vi "HXQ-钩外多胶-检测.vi"(5 "裁切偏移":i32[](array[numeric]), 7 "ImgRef":T8(plugin-control), 9 "MirroredAngle":dbl, 10 "Global Rectangle":i32[](array[numeric]), 11 "ImageSRC":T8(plugin-control)) -> (0 "顶洞缺胶状态正常":bool, 1 "多胶异常RECT":cluster{dbl, dbl, dbl, dbl}, 2 "钩外多胶正常":bool, 3 "ImageOUT":T8(plugin-control))   [LabVIEW 2018]
uses:
  <vilib>/vision/Measure.llb/Straight Edge Options.ctl
  <vilib>/vision/Measure.llb/Straight Edge Process.ctl
  <vilib>/vision/Measure.llb/Edge Options.ctl
  <vilib>/vision/Measure.llb/Edge Polarity.ctl
  <vilib>/vision/Image Controls.llb/IMAQ Image.ctl
  <vilib>/vision/Contour.llb/IMAQ Contour Curve Extraction.ctl
  <vilib>/Analysis/coordinate.llb/Angle Units.ctl
  <vilib>/Analysis/coordinate.llb/Check for Included Angle (scalar).vi
  <vilib>/Analysis/coordinate.llb/Wrap Angle (scalar).vi
  <vilib>/Analysis/coordinate.llb/Absolute Angle Difference (scalar).vi
  <vilib>/Analysis/coordinate.llb/Set Angle Unit.vi
  <vilib>/vision/NI_Vision_Development_Module.lvlib
  <vilib>/Analysis/NI_AAL_Angle.lvlib
  <vilib>/vision/Contour.llb/IMAQ Connect Range Setting.ctl
panel:
  in  "Contour Points Settings":T1={"Overlay?"=TRUE, "Color"=16738816, "Width"=1, "Maintain Width?"=TRUE}
  in  "Kernel Width":u32=31
  in  "Curve Extraction Settings":T2={"Extraction Mode"=0, "Edge Threshold"=30, "Edge Filter Size"=2, "Min Length"=10, "Search Step Size"=10, "Max Endpoint Gap"=20, "Subpixel"=TRUE} {"Extraction Mode" items=["Normal", "Uniform Regions"]; "Edge Filter Size" items=["Fine", "Normal", "Contour Tracing"]; "Max Endpoint Gap" min=0; "Search Step Size" min=1 max=255 step=1; "Min Length" min=0; "Edge Threshold" min=1 max=350 step=1}
  out "Curvature Profile":dbl[](graph)
  in  "顶洞_RakeEdge Options 2":T3={"Edge Polarity"=0, "Kernel Size"=3, "Width"=9, "Minimum Edge Strength"=50.0, "Interpolation Type"=enum."Bilinear Fixed", "Data Processing Method"=enum."Average"} {"Edge Polarity" items=["All Edges", "Rising Edges", "Falling Edges"]; "Minimum Edge Strength" format="%.2f"; "Width" step=2; "Kernel Size" step=2}
  out "顶洞圆半径正常":bool
  out "顶洞圆半径":dbl
  in  "顶洞圆半径下限":dbl=50.0
  in  "顶洞圆半径上限":dbl=330.0
  out "Fitted Circle":T5 {"Average SNR (dB)" format="%.2f"; "Average Strength" format="%.2f"; "Roundness (Real-World)" format="%.2f"; "Radius (Real-World)" format="%.2f"; "Center (Real-World)"."Y" format="%.2f"; "Center (Real-World)"."X" format="%.2f"; "Radius (Pixels)" format="%.2f"; "Center (Pixels)"."Y" format="%.2f"; "Center (Pixels)"."X" format="%.2f"}
  in  "顶洞_Options":T6={"Search  Direction"=0, "Edge Options"={"Edge Polarity"=0, "Kernel Size"=3, "Width"=9, "Minimum Edge Strength"=50.0, "Interpolation Type"=enum."Bilinear Fixed", "Data Processing Method"=enum."Average"}, "Show Search Area"=TRUE, "Show Search Lines"=FALSE, "Show Edges Found"=FALSE, "Show Result"=TRUE, "Search Area Color"=65280, "Search Lines Color"=255, "Edge Locations Color"=16776960, "Result Color"=16711680, "Overlay Group Name"=""} {"Search  Direction" items=["Outside to Inside", "Inside to Outside"]; "Edge Options"."Edge Polarity" items=["All Edges", "Rising Edges", "Falling Edges"]; "Edge Options"."Minimum Edge Strength" format="%.2f"; "Edge Options"."Width" step=2; "Edge Options"."Kernel Size" step=2}
  in  "顶洞_Circle Fit Options":T7={"Process"=enum."Get First Edge", "Step Size"=3.0, "Max Pixel Radius"=3}
  in  "ROI_顶洞检测扇形半张角":dbl=17.0 format="%#_13g"
  in  "R_顶洞检测小圆半径":i32=136
  out "ImgOut":T8(plugin-control)
  in  "偏移_顶洞_向上部修正量":dbl=230.0 format="%#_13g"
  in  "槽宽比例限度":dbl=0.04
  out "多胶异常RECT本地":T9
  out "error out 2":errorcluster
  out "Image Out":T8
  in  "偏移_钩端_向上部修正量":dbl=209.0 format="%#_13g"
  in  "初始ROI下行参数":dbl=1.0
  in  "高径比参数值":dbl=0.6
  out "边沿检测LineProfile原始":dbl[](graph)
  out "波形2":dbl[](graph) caption="Line Profile"
  out "边沿检测梯度":dbl[](graph)
  in  "溢槽槽向边沿检测":T3={"Edge Polarity"=1, "Kernel Size"=7, "Width"=37, "Minimum Edge Strength"=50.0, "Interpolation Type"=enum."Bilinear Fixed", "Data Processing Method"=enum."Average"} {"Edge Polarity" items=["All Edges", "Rising Edges", "Falling Edges"]; "Minimum Edge Strength" format="%.2f"; "Width" step=2; "Kernel Size" step=2}
  out "所得中线的端点属于正序":bool caption="范围内？"
  out "Angles (deg)":sgl[](array[numeric]) format="%.2f"
  out "error out":errorcluster
  in  "error in (no error)":errorcluster
  in  "Image":T8
  in  "Edge Options横向槽边":T3={"Edge Polarity"=2, "Kernel Size"=7, "Width"=13, "Minimum Edge Strength"=70.0, "Interpolation Type"=enum."Bilinear Fixed", "Data Processing Method"=enum."Average"} {"Edge Polarity" items=["All Edges", "Rising Edges", "Falling Edges"]; "Minimum Edge Strength" format="%.2f"; "Width" step=2; "Kernel Size" step=2}
  in  "Line Options":T10={"Number of Lines"=1, "Type"=enum."First Edge Rake", "Min. Score"=100.0, "Max. Score"=1000.0, "Orientation"=0.0, "Angle Range"=10.0, "Angle Tolerance"=1.0, "Step Size"=5, "Min. SNR (db)"=0.0, "Min. Points (%)"=25.0, "Hough Iterations"=5} {"Min. Points (%)" min=0.0 max=100.0; "Min. SNR (db)" min=0.0; "Max. Score" min=0.0 max=1024.0; "Min. Score" min=0.0 max=1024.0 step=1.0}
  # "小洞，大洞：50,110"
  # "进行槽的横向边沿检测的时候\n最好对强度阈值进行动态自动配置，避免定值"
  # "槽的边沿强度需要认真设定，避免强度门槛太低引入干扰致找错位置。"
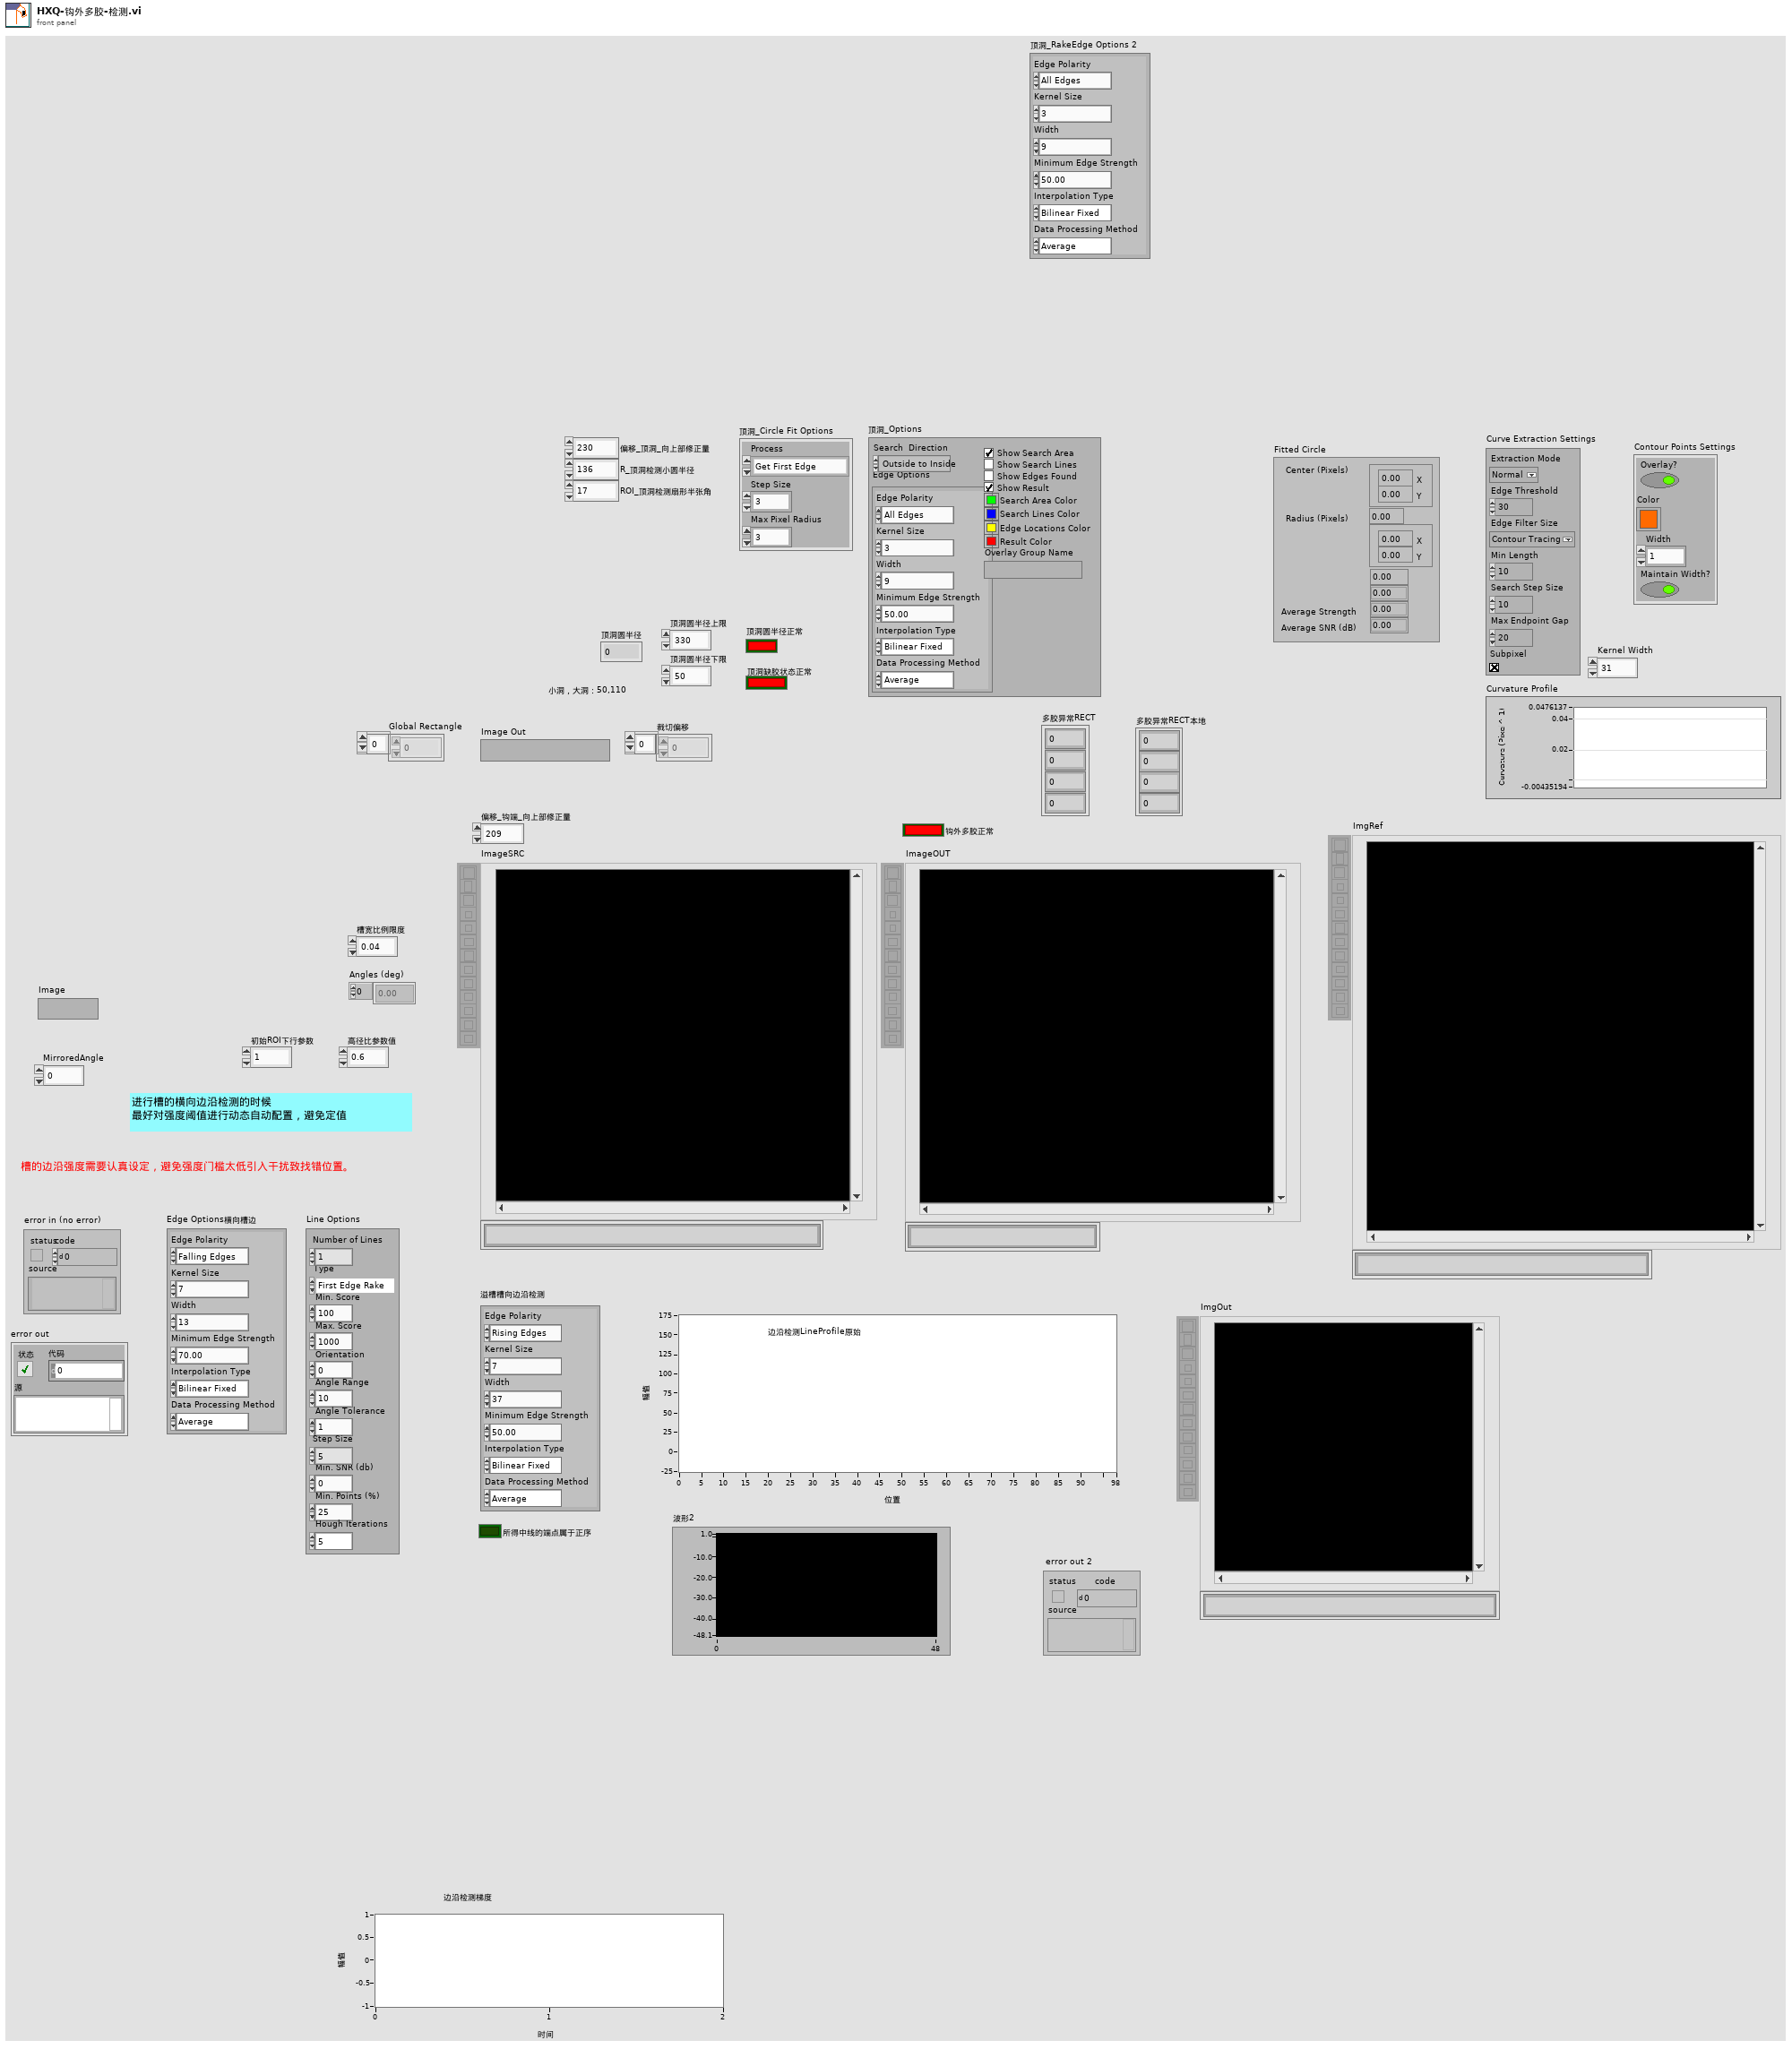
[diagram p1: front panel]
types:
  T1 = cluster{"Overlay?":bool, "Color":u32, "Width":u32, "Maintain Width?":bool}
  T2 = typedef "IMAQ Contour Curve Extraction.ctl" = cluster{"Extraction Mode":u32, "Edge Threshold":i32, "Edge Filter Size":u32, "Min Length":i32, "Search Step Size":i32, "Max Endpoint Gap":i32, "Subpixel":bool}
  T3 = typedef "Edge Options.ctl" = cluster{"Edge Polarity":T4, "Kernel Size":u32, "Width":u32, "Minimum Edge Strength":sgl, "Interpolation Type":enum32{"Zero Order", "Bilinear", "Quadratic", "Cubic", "Bilinear Fixed"}, "Data Processing Method":enum32{"Average", "Median"}}
  T4 = typedef "Edge Polarity.ctl" = u32
  T5 = cluster{"Center (Pixels)":cluster{"X":sgl, "Y":sgl}, "Radius (Pixels)":dbl, "Center (Real-World)":cluster{"X":sgl, "Y":sgl}, "Radius (Real-World)":dbl, "Roundness (Real-World)":dbl, "Average Strength":dbl, "Average SNR (dB)":dbl}
  T6 = cluster{"Search  Direction":u32, "Edge Options":T3, "Show Search Area":bool, "Show Search Lines":bool, "Show Edges Found":bool, "Show Result":bool, "Search Area Color":u32, "Search Lines Color":u32, "Edge Locations Color":u32, "Result Color":u32, "Overlay Group Name":string}
  T7 = cluster{"Process":enum16{"Get First Edge", "Get First + Last Edge", "Get All Edges", "Get Best Edge"}, "Step Size":dbl, "Max Pixel Radius":i32}
  T8 = typedef "IMAQ Image.ctl" = refnum<image>
  T9 = cluster{"Numeric":dbl, "Numeric":dbl, "Numeric":dbl, "Numeric":dbl}
  T10 = typedef "Straight Edge Options.ctl" = cluster{"Number of Lines":i32, "Type":T11, "Min. Score":dbl, "Max. Score":dbl, "Orientation":dbl, "Angle Range":dbl, "Angle Tolerance":dbl, "Step Size":u32, "Min. SNR (db)":dbl, "Min. Points (%)":dbl, "Hough Iterations":i32}
  T11 = typedef "Straight Edge Process.ctl" = enum32{"First Edge Rake", "Best Edge Rake", "Hough Edge Rake", "First Edge Projection", "Best Edge Projection"}
  T12 = typedef "IMAQ Point" = cluster{"X":sgl, "Y":sgl}
  T13 = enum16{"Get First Edge", "Get First + Last Edge", "Get All Edges", "Get Best Edge"}
  T14 = typedef "ROI Descriptor" = cluster{"Global Rectangle":i32[], "Contours":cluster{"ID":enum32{"External", "Internal"}, "Type":u32, "Coordinates":i32[]}[]}
  T15 = cluster{"X":dbl, "Y":dbl, "X":dbl, "Y":dbl, "Height":dbl}
  T16 = typedef "Edge New.ctl" = cluster{"Location (Pixel)":cluster{"X":sgl, "Y":sgl}, "Location (Real-World)":cluster{"X":sgl, "Y":sgl}, "Distance (Pixel)":dbl, "Distance (Real-World)":dbl, "Strength":dbl, "Noise":dbl, "Rising?":bool}
  T17 = typedef "Search Line.ctl" = cluster{"Start Point":cluster{"X":sgl, "Y":sgl}, "End Point":cluster{"X":sgl, "Y":sgl}, "Edge Info":T16[], "Edge Map":dbl[], "Calibration Valid":bool}
  T18 = cluster{"Point1 (Pixels)":cluster{"X":sgl, "Y":sgl}, "Point2 (Pixels)":cluster{"X":sgl, "Y":sgl}, "Point1 (Real-World)":cluster{"X":sgl, "Y":sgl}, "Point2 (Real-World)":cluster{"X":sgl, "Y":sgl}, "Angle (Pixel)":dbl, "Angle (Real-World)":dbl, "Score":dbl, "Straightness":dbl, "Average SNR (db)":dbl, "Calibration Valid":bool}[]
  T19 = cluster{"Point1 (Pixels)":cluster{"X":sgl, "Y":sgl}, "Point2 (Pixels)":cluster{"X":sgl, "Y":sgl}, "Point1 (Real-World)":cluster{"X":sgl, "Y":sgl}, "Point2 (Real-World)":cluster{"X":sgl, "Y":sgl}, "Angle (Pixel)":dbl, "Angle (Real-World)":dbl, "Score":dbl, "Straightness":dbl, "Average SNR (db)":dbl, "Calibration Valid":bool}
  T20 = cluster{"Point2 (Pixels)":cluster{"X":sgl, "Y":sgl}, "Point1 (Pixels)":cluster{"X":sgl, "Y":sgl}}
  T21 = typedef "IMAQ Line" = cluster{"Start X":i32, "Start Y":i32, "End X":i32, "End Y":i32}
  T22 = typedef "IMAQ Circle" = cluster{"Center X":i32, "Center Y":i32, "Inner Radius":i32, "Outer Radius":i32, "Start Angle":dbl, "End Angle":dbl}
  T23 = typedef "IMAQ Connect Range Setting.ctl" = cluster{"Match Constraints":u32, "Min":dbl, "Max":dbl}
  T24 = enum16{"Closest To Search Start", "Maximum Length", "Strongest Mean Gradient Change"}
  T25 = enum16{"Rect Left To Right", "Rect Right To Left", "Rect Top To Bottom", "Rect Bottom To Top", "Annulus Inner To Outer", "Annulus Outer To Inner", "Annulus Start Angle To End Angle", "Annulus End Angle To Start Angle"}
  T26 = typedef "IMAQ Rectangle" = cluster{"Left":i32, "Top":i32, "Right":i32, "Bottom":i32, "Rotation":dbl}
  T27 = typedef "NI_AAL_Angle.lvlib/Angle Units.ctl" = i32
  T28 = cluster{"Point1 (Pixels)":cluster{"X":sgl, "Y":sgl}, "Point2 (Pixels)":cluster{"X":sgl, "Y":sgl}}
  T29 = cluster{"Point 1":cluster{"X":sgl, "Y":sgl}, "Point 2":cluster{"X":sgl, "Y":sgl}}
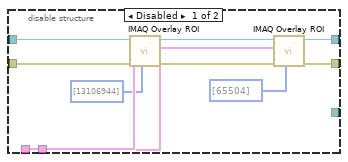
[diagram p4: hidden frame]
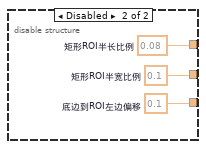
[diagram p5: hidden frame]
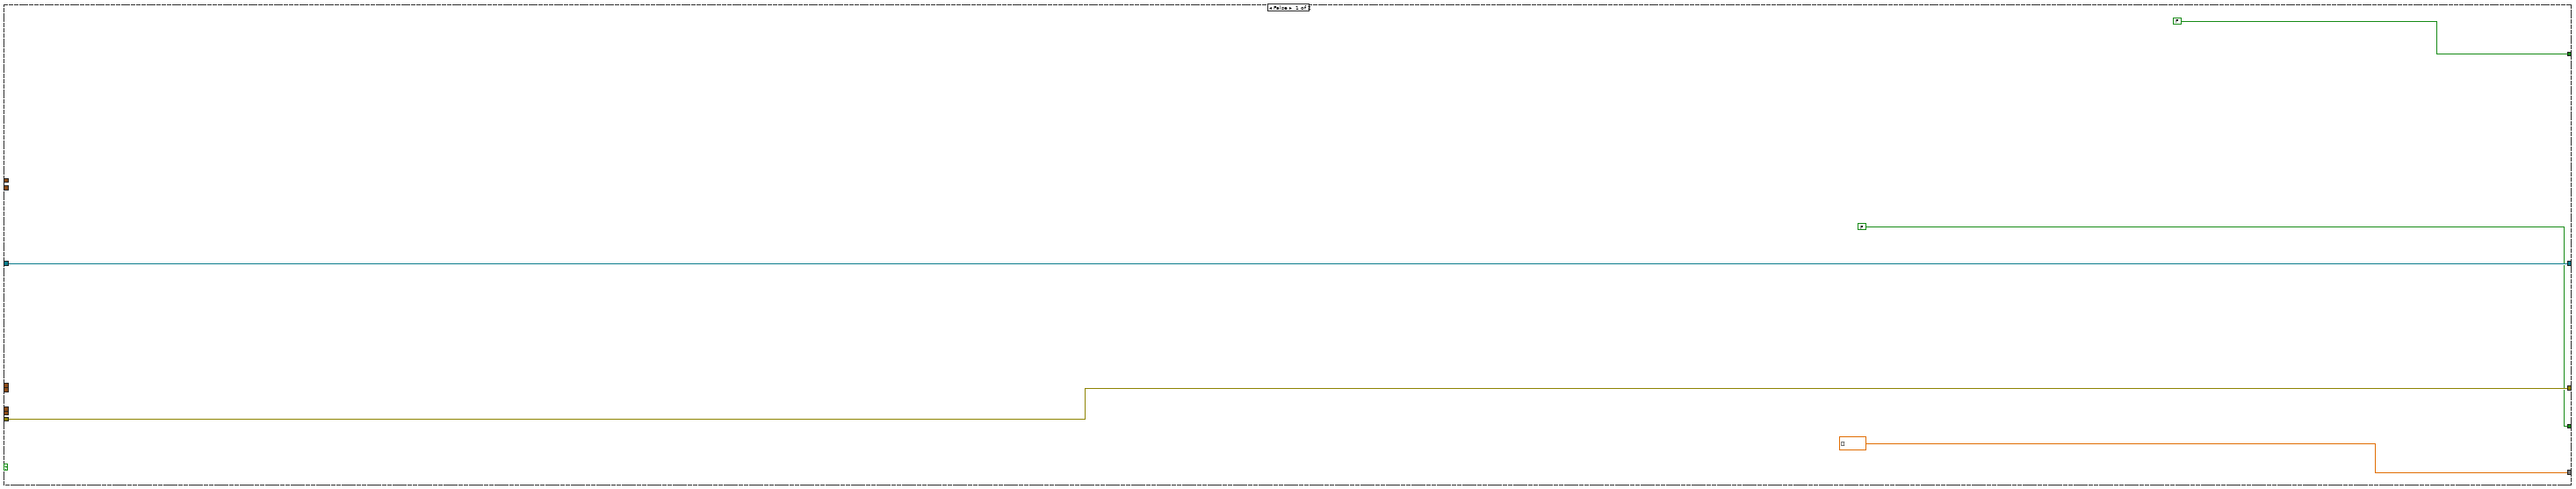
[diagram p13: hidden frame]
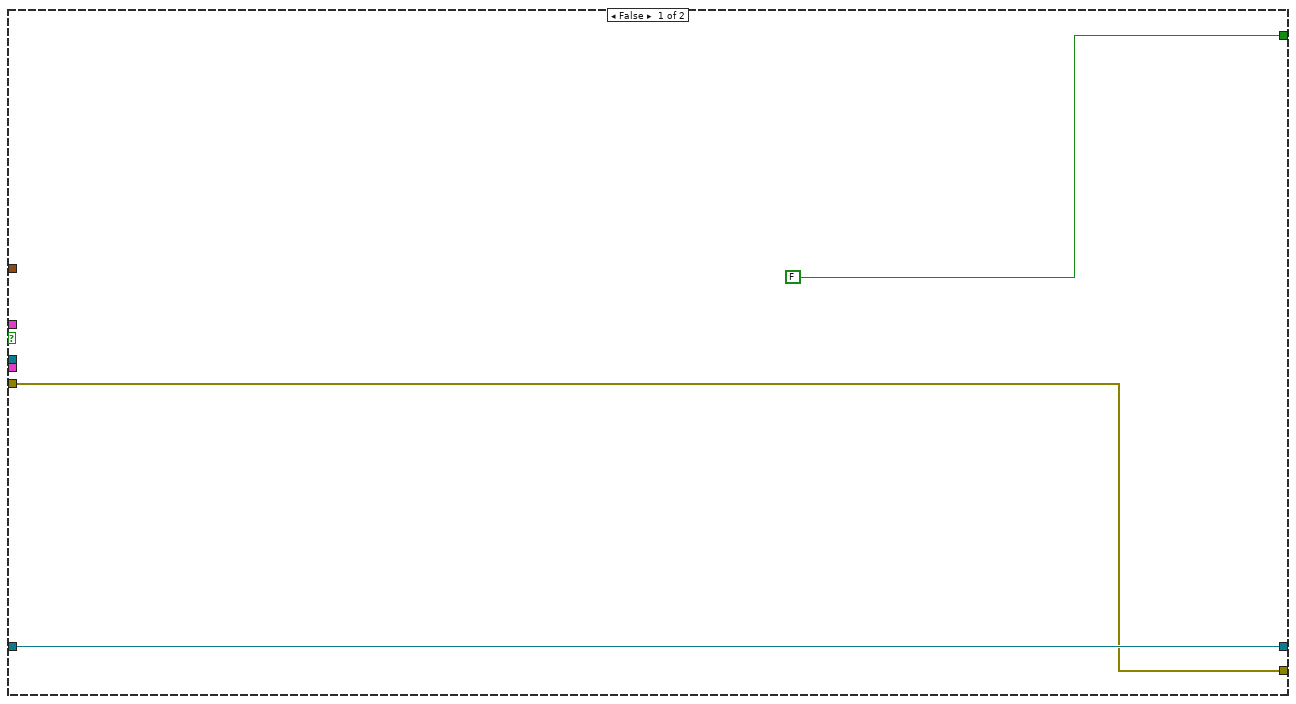
[diagram p14: hidden frame]
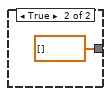
[diagram p19: hidden frame]
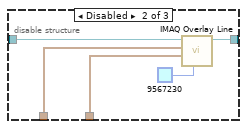
[diagram p20: hidden frame]
diagram:
  w1 = TRUE ("顶洞缺胶状态正常")
  w68 = T12 {"X"=0.5, "Y"=0.5}  # 中点比例
  w83 = 0.1  # 底边到ROI左边偏移
  w81 = 0.15  # 矩形ROI半宽比例
  w80 = 0.05  # 矩形ROI半长比例
  w88 = 0.5 ("y")
  w143 = 0.5 ("y")
  w124 = -0.05  # 底边到ROI左边偏移
  w123 = 0.03  # 矩形ROI半宽比例
  w122 = 0.1  # 矩形ROI半长比例
  # "获取槽位的边沿强度，\n用以指导随后的边线搜索时边沿强度阈值"
  # "经验值"
  # "注意：如果外部裁切时遇到边界，则裁切的XY尺寸会发生异常，\n不能代表产品的半径，导致定位异常。"
  # "构建ROI用于检测铜底最低点"
  # "找寻铜底最低处的位置\n给出准确的基准用于划定扇形ROI选出钩端区域"
  # "从大图中截取时，适当留出边际，以免检测底沿时遇到图像边界。"
  # "矩形ROI的大小，最好改为与底圆直径挂钩，以免后期调节（已挂钩）"
  n1 = disable-structure shown="启用" {
    disable-tunnel: [w169 w172] -> w163
    disable-tunnel: [w168 w171] -> w162
    disable-tunnel: [w167 w170] -> w161
    frame Enabled {
      w167 = 0.06  # 底边到ROI左边偏移
      w168 = 0.11  # 矩形ROI半宽比例
      w169 = 0.15  # 矩形ROI半长比例
    }
    frame Disabled {
      w170 = 0.1  # 底边到ROI左边偏移
      w171 = 0.1  # 矩形ROI半宽比例
      w172 = 0.08  # 矩形ROI半长比例
    }
  }
  n2 = call "IMAQ Clear Overlay"("Image"="ImgRef") -> ("error out"=w125:errorcluster, "Image Out"=w115:T8)  [unwired: 9 in]
  n3 = call "IMAQ GetImageSize"("Image"=w115, "error in (no error)"=w125) -> ("Y Resolution"=w129:i32, "X Resolution"=w130:i32, "error out"=w128:errorcluster)  [unwired: 2 in]
  n4 = Multiply(x=w130, y=w143) -> (x*y=w140:dbl)
  n5 = Multiply(x=w129, y=w143) -> (x*y=w144:dbl)
  n6 = call "IMAQ GetImageSize"("Image"="ImageSRC", "error in (no error)"="error in (no error)") -> ("Y Resolution"=w84:i32, "X Resolution"=w33:i32, "error out"=w27:errorcluster)  [unwired: 2 in]
  n7 = call "HXQ-局部-创建特征检测矩形区域A.vi"("方向角"="MirroredAngle", "产品参考半径"=w33, "底边到ROI左边偏移"=w161, "高径比参数值"="高径比参数值", "矩形ROI半宽比例"=w162, "矩形ROI半长比例"=w163, "Y Resolution"=w84, "X Resolution"=w33) -> ("矩形输出"=w17:cluster{dbl, dbl, dbl, dbl, dbl})  [unwired: 1 in, 2 out]
  n8 = Bundle(w140, w144) -> (w142:cluster{dbl, dbl})  [unwired: 1 in]
  n9 = call "HXQ-局部-创建特征检测矩形区域A.vi"("方向角"="MirroredAngle", "产品参考半径"=w33, "底边到ROI左边偏移"=w83, "矩形ROI半宽比例"=w81, "矩形ROI半长比例"=w80, "Y Resolution"=w84, "X Resolution"=w33) -> ("Height"=w47:dbl, "矩形输出"=w79:cluster{dbl, dbl, dbl, dbl, dbl})  [unwired: 2 in, 1 out]
  n10 = Random Number (0-1)() -> (number: 0 to 1=w11:dbl)
  n11 = call "HXQ-局部-创建特征检测矩形区域A.vi"("方向角"="MirroredAngle", "产品参考半径"=w33, "底边到ROI左边偏移"=w124, "高径比参数值"="高径比参数值", "矩形ROI半宽比例"=w123, "矩形ROI半长比例"=w122, "Y Resolution"=w129, "X Resolution"=w130) -> ("矩形输出"=w160:cluster{dbl, dbl, dbl, dbl, dbl})  [unwired: 1 in, 2 out]
  n12 = Multiply(x=w11, y=100000000.0) -> (x*y=w12:dbl)
  n13 = call "IMAQ Clear Overlay"("error in (no error)"=w27, "Image"="ImageSRC") -> ("error out"=w66:errorcluster, "Image Out"=w67:T8)  [unwired: 8 in]
  n14 = To Unsigned Long Integer(number=w12) -> (unsigned 32bit integer=w15:u32)
  n15 = call "IMAQ Convert Rectangle to ROI (Polygon)"("Rectangle"=w79) -> ("error out"=w26:errorcluster, "Rectangle Points"=w76:T12[])  [unwired: 7 in, 1 out]
  n16 = Index Array(array=w76, index #1=0 ("索引"), index #2=1 ("索引"), index #3=2 ("索引"), index #4=3 ("索引")) -> (element #1=w51:T12, element #2=w71:T12, element #3=w50:T12, element #4=w49:T12)
  n17 = disable-structure shown="禁用" {
    frame Disabled {
      w175 = cluster{"X":sgl, "Y":sgl} {"X"=10.0, "Y"=10.0} ("y")
      n18 = Add(x=w175, y=cluster{"X":sgl, "Y":sgl} {"X"=1.0, "Y"=0.0}) -> (x+y=w179:cluster{"X":sgl, "Y":sgl})
      n19 = Build Array(w179, cluster{"X":sgl, "Y":sgl} {"X"=15.0, "Y"=5.0} ("y")) -> (w178:cluster{"X":sgl, "Y":sgl}[])
      n20 = call "IMAQ Get Angles"("Vertex"=w175, "Points"=w178, "Use Vertex (No)"=TRUE) -> ("Angles (deg)"=→"Angles (deg)":sgl[])  [unwired: 2 in, 2 out]
    }
    frame Enabled {
    }
  }
  n21 = Number To Hexadecimal String(2:w15) -> (0:w13:string)  [unwired: 1 in]
  n22 = call "IMAQ Convert Rectangle to ROI (Polygon)"("error in (no error)"=w128, "Rectangle"=w160) -> ("error out"=w156:errorcluster, "ROI Descriptor"=w146:T14)  [unwired: 6 in, 1 out]
  n23 = Subtract(x=w51, y=w49) -> (x-y=w48:T12)
  n24 = Concatenate Strings("HXQGWDJ_GREYEDGE1" ("字符串"), w13) -> (w14:string)
  n25 = Add(x=w51, y=w71) -> (x+y=w70:T12)
  n26 = Add(x=w50, y=w49) -> (x+y=w69:T12)
  n27 = Divide(x=w48, y=w47) -> (x/y=w46:cluster{"X":dbl, "Y":dbl})
  n28 = Multiply(x=w70, y=w68) -> (x*y=w65:T12)
  n29 = Multiply(x=w69, y=w68) -> (x*y=w60:T12)
  n30 = call "IMAQ Create"("Image Name"=w14) -> ("New Image"=w5:T8)  [unwired: 4 in, 1 out]
  n31 = Multiply(x=w46, y=20.0 ("Height")) -> (x*y=w44:cluster{"X":dbl, "Y":dbl})
  n32 = Unbundle(w65) -> ("X"=w64:sgl, "Y"=w63:sgl)
  n33 = Unbundle(w60) -> ("X"=w62:sgl, "Y"=w61:sgl)
  n34 = Unbundle(w44) -> ("X"=w43:dbl, "Y"=w42:dbl)
  n35 = Bundle("X"=w64, "Y"=w63, "X"=w62, "Y"=w61) -> (w59:cluster{"X":sgl, "Y":sgl, "X":sgl, "Y":sgl})  [unwired: 1 in]
  n36 = Bundle("X"=w43, "Y"=w42, "X"=w43, "Y"=w42, "Height"=0.0) -> (w40:T15)  [unwired: 1 in]
  n37 = Multiply(x=w33, y=w88) -> (x*y=w89:dbl)
  n38 = Multiply(x=w84, y=w88) -> (x*y=w87:dbl)
  n39 = call "IMAQ Convert Line to ROI"("error in (no error)"=w26, "Line"=w59) -> ("error out"=w25:errorcluster, "ROI Descriptor"=w38:T14)  [unwired: 7 in]
  n40 = Bundle "图像中心点"(w89, w87) -> (w86:cluster{dbl, dbl})  [unwired: 1 in]
  n41 = call "IMAQ Rake 3"("Image"=w115, "Edge Options"=T3 {"Edge Polarity"=2, "Kernel Size"=5, "Width"=45, "Minimum Edge Strength"=30.0, "Interpolation Type"=enum."Bilinear Fixed", "Data Processing Method"=enum."Average"}, "Optimized Mode"=TRUE, "ROI Descriptor"=w146, "Step Size"=u32 5, "error in (no error)"=w156, "Process"=T13."Get First Edge") -> ("First Edges"=w133:T16[], "Search Lines"=w137:T17[], "error out"=w127:errorcluster)  [unwired: 5 in, 1 out]
  n42 = Add(x=w17, y=w40) -> (x+y=w39:cluster{dbl, dbl, dbl, dbl, dbl})
  n43 = Subtract(x=w17, y=w40) -> (x-y=w31:cluster{dbl, dbl, dbl, dbl, dbl})
  n44 = call "IMAQ Edge Tool 3"("Image"=w67, "Edge Options"="Edge Options横向槽边", "Optimized Mode"=FALSE, "ROI Descriptor"=w38) -> ("Image (duplicate)"=w6:T8, "Gradient Values"=w57:dbl[], "error out"=w30:errorcluster)  [unwired: 7 in, 2 out]
  n45 = Array Max & Min(array=w57) -> (max value=w56:dbl)  [unwired: 3 out]
  n46 = call "IMAQ Convert Rectangle to ROI (Polygon)"("Rectangle"=w17) -> ("ROI Descriptor"=w21:T14)  [unwired: 7 in, 2 out]
  n47 = call "IMAQ Convert Rectangle to ROI (Polygon)"("Rectangle"=w39) -> ("error out"=w29:errorcluster, "ROI Descriptor"=w20:T14)  [unwired: 7 in, 1 out]
  n48 = call "IMAQ Convert Rectangle to ROI (Polygon)"("error in (no error)"=w25, "Rectangle"=w31) -> ("error out"=w28:errorcluster, "ROI Descriptor"=w19:T14)  [unwired: 6 in, 1 out]
  n49 = call "IMAQ Overlay ROI"("Colors (Green)"=u32[] [16775680], "error in (no error)"=w66, "ROI Descriptor"=w38, "Image"=w67) -> ("error out"=w77:errorcluster, "Image Out"=w78:T8)  [unwired: 6 in]
  n50 = Empty Array?(array=w133) -> (empty?=w132:bool)
  n51 = call "IMAQ Overlay ROI"("Colors (Green)"=u32[] [9567230], "error in (no error)"=w127, "ROI Descriptor"=w146, "Image"=w115) -> ("error out"=w111:errorcluster, "Image Out"=w113:T8)  [unwired: 6 in]
  n52 = disable-structure shown="禁用" {
    disable-tunnel: w137 -> [w182 _]
    frame Disabled {
      n53 = Index Array(array=w182) -> (element=w181:T17)  [unwired: 1 in]
      n54 = Unbundle By Name(w181) -> ("Edge Map"=→"波形2":dbl[])
    }
    frame Enabled {
    }
  }
  n55 = Multiply(x=w56, y=0.5) -> (x*y=w52:dbl)
  n56 = Bundle By Name(cluster="Edge Options横向槽边", "Minimum Edge Strength"=w52) -> (w53:T3)
  n57 = for {
    tunnel: w133 -> [w185] mode=indexing
    tunnel: [w184] -> w151 mode=indexing
    tunnel: [w183] -> w153 mode=indexing
    n58 = Unbundle By Name(w185) -> ("Location (Pixel)"=w184:cluster{"X":sgl, "Y":sgl}, "Distance (Pixel)"=w183:dbl)
  }
  n59 = Build Array(w21, w20, w19) -> (w18:T14[])
  n60 = Merge Errors(w30, w29, w28) -> (w3:errorcluster)
  n61 = call "提取G分量"("Image In"=w6, "Image Dst"=w5, "error in"=w3) -> ("Image Out"=w4:T8, "error out"=w2:errorcluster)  [unwired: 23 in]
  n62 = Array Max & Min(array=w153) -> (min index (indices)=w152:i32)  [unwired: 3 out]
  n63 = Index Array(array="裁切偏移", index #1=0 ("索引"), index #2=1 ("索引")) -> (element #1=w118:i32, element #2=w117:i32)
  n64 = Index Array(array=w151, index=w152) -> (element=w108:cluster{"X":sgl, "Y":sgl})
  n65 = Build Array(w108) -> (w109:cluster{"X":sgl, "Y":sgl}[])
  n66 = call "Overlay Feature Points.vi"("Color"=u32 16860, "error in"=w111, "Feature Points"=w109, "Image"=w113) -> ("error out"=→"error out 2":errorcluster, "Image Out"=→"Image Out":T8)  [unwired: 6 in]
  n67 = Bundle(w118, w117) -> (w116:cluster{i32, i32})  [unwired: 1 in]
  n68 = for {
    tunnel: w53 -> [w214]
    tunnel: [w206] -> w37
    tunnel: [w207] -> w36
    tunnel: [w208] -> w35
    tunnel: [w204] -> w34
    shift-right: [w190] -> w8
    shift-left: w2 -> [w215]
    tunnel: w33 -> [w201]
    tunnel: [w195] -> w32
    shift-right: [w188] -> w22
    shift-left: w6 -> [w194]
    tunnel: w18 -> [w189] mode=indexing
    tunnel: [w187] -> w9
    tunnel: w4 -> [w186]
    stop <- w195 continue-if-true
    w211 = 0 ("索引")
    w218 = u32 3 items=["Left to Right", "Right to Left", "Top to Bottom", "Bottom to Top"] ("Search Direction")
    w219 = u32 2 items=["Left to Right", "Right to Left", "Top to Bottom", "Bottom to Top"] ("Search Direction")
    # "计算其中一条线端点到另一条线的距离\n评估线间距的合规程度"
    n69 = call "IMAQ Overlay ROI"("Colors (Green)"=u32[] [65280], "ROI Descriptor"=w189, "Image"=w194) -> ("Image Out"=w188:T8)  [unwired: 7 in, 1 out]
    n70 = call "IMAQ Find Straight Edges 3"("Image"=w186, "Edge Options"=w214, "ROI Descriptor"=w189, "Search Direction"=w219, "error in (no error)"=w215, "Line Options"="Line Options") -> ("Image (duplicate)"=w193:T8, "Straight Edges"=w210:T18, "error out"=w216:errorcluster)  [unwired: 5 in, 2 out]
    n71 = call "IMAQ Find Straight Edges 3"("Image"=w193, "Edge Options"=w214, "ROI Descriptor"=w189, "Search Direction"=w218, "error in (no error)"=w216, "Line Options"="Line Options") -> ("Image (duplicate)"=w187:T8, "Straight Edges"=w209:T18, "error out"=w203:errorcluster)  [unwired: 5 in, 2 out]
    n72 = Empty Array?(array=w210) -> (empty?=w198:bool)
    n73 = Empty Array?(array=w209) -> (empty?=w197:bool)
    n74 = Index Array(array=w210, index=w211) -> (element=w213:T19)
    n75 = Index Array(array=w209, index=w211) -> (element=w212:T19)
    n76 = Unbundle By Name(w213) -> ("Point1 (Pixels)"=w206:cluster{"X":sgl, "Y":sgl}, "Point2 (Pixels)"=w207:cluster{"X":sgl, "Y":sgl})
    n77 = Unbundle By Name(w212) -> ("Point1 (Pixels)"=w208:cluster{"X":sgl, "Y":sgl}, "Point2 (Pixels)"=w204:cluster{"X":sgl, "Y":sgl})
    n78 = Bundle("Point2 (Pixels)"=w207, "Point1 (Pixels)"=w206) -> (w205:T20)  [unwired: 1 in]
    n79 = Multiply(x=w201, y="槽宽比例限度") -> (x*y=w199:dbl)
    n80 = call "IMAQ Perpendicular Line"("error in (no error)"=w203, "Point"=w204, "Line"=w205) -> ("error out"=w191:errorcluster, "Distance"=w202:dbl)  [unwired: 6 in, 1 out]
    n81 = Greater?(x=w202, y=w199) -> (0:w196:bool)
    n82 = call <vilib>:"Clear Errors.vi"("error in (no error)"=w191) -> ("error out"=w190:errorcluster)  [unwired: 5 in, 1 out]
    n83 = Compound Arithmetic op=OR ("复合运算")(w196, w198, w197) -> (w195:bool)
  }
  n84 = disable-structure shown="启用" {
    disable-tunnel: w78 -> [w229 _]
    disable-tunnel: w77 -> [w228 w231]
    disable-tunnel: _ -> [w227 _]
    disable-tunnel: [w225 w230] -> w24
    disable-tunnel: [w223 w231] -> w23
    disable-tunnel: _ -> [w221 _]
    disable-tunnel: w22 -> [_ w230]
    frame Disabled {
      n85 = call "IMAQ Overlay ROI"("Colors (Green)"=u32[] [13106944], "error in (no error)"=w228, "ROI Descriptor"=w227, "Image"=w229) -> ("error out"=w224:errorcluster, "Image Out"=w226:T8)  [unwired: 6 in]
      n86 = call "IMAQ Overlay ROI"("Colors (Green)"=u32[] [65504], "error in (no error)"=w224, "ROI Descriptor"=w221, "Image"=w226) -> ("error out"=w223:errorcluster, "Image Out"=w225:T8)  [unwired: 6 in]
    }
    frame Enabled {
    }
  }
  n87 = Add(x=w108, y=w116) -> (x+y=w85:cluster{sgl, sgl})
  n88 = Build Array(w142, w108) -> (w145:cluster{"X":dbl, "Y":dbl}[])
  n89 = Build Array(w85) -> (w148:cluster{sgl, sgl}[])
  n90 = call "IMAQ Point Distances"("Points"=w145) -> ("Distances"=w141:sgl[])  [unwired: 4 in, 1 out]
  n91 = call "Overlay Feature Points.vi"("Color"=u32 16860, "error in"=w23, "Feature Points"=w148, "Image"=w24) -> ("error out"=w135:errorcluster, "Image Out"=w149:T8)  [unwired: 6 in]
  n92 = Index Array(array=w141) -> (element=w139:sgl)  [unwired: 1 in]
  n93 = call "IMAQ Dispose"("Image"=w9, "error in (no error)"=w8) -> ("error out"=w7:errorcluster)  [unwired: 4 in]
  n94 = Compound Arithmetic op=OR ("复合运算")(w132, w32) -> (w136:bool)
  n95 = Merge Errors(w135, w7) -> (w134:errorcluster)
  n96 = case shown="假" w136 {
    tunnel: w149 -> [w248 w590]
    tunnel: [w260 w590] -> w164
    tunnel: w134 -> [w257 w589]
    tunnel: [w251 w589] -> w165
    tunnel: "MirroredAngle" -> [w250 _]
    tunnel: [w241 FALSE] -> w90
    tunnel: w139 -> [w240 _]
    tunnel: [w239 dbl[] [] ("Particle Measurements (Pixels) (Particle Analysis 1)")] -> w97
    tunnel: w86 -> [w238 _]
    tunnel: w85 -> [w237 _]
    tunnel: w37 -> [w236 _]
    tunnel: w36 -> [w235 _]
    tunnel: w35 -> [w234 _]
    tunnel: w34 -> [w233 _]
    tunnel: [w232 FALSE] -> _
    frame False {
      w245 = u32 16860 ("Color")
      w242 = sgl 8.0  # 夹角允许值
      # "合规：夹角小于特定值"
      # "计算槽中分线"
      n97 = call "IMAQ Overlay Line"("Color"=w245, "End Point"=w234, "Start Point"=w233, "Image"=w248) -> ("error out"=w246:errorcluster, "Image Out"=w247:T8)  [unwired: 6 in]
      n98 = Build Array "确认边沿夹角正常"(w236, w235, w234, w233) -> (w261:cluster{"X":sgl, "Y":sgl}[])
      n99 = call "IMAQ Get Angles"("error in (no error)"=w257, "Points"=w261) -> ("error out"=w252:errorcluster, "Angles (deg)"=w259:sgl[])  [unwired: 3 in, 1 out]
      n100 = call "IMAQ Overlay Line"("Color"=w245, "error in (no error)"=w246, "End Point"=w236, "Start Point"=w235, "Image"=w247) -> ("Image Out"=w249:T8)  [unwired: 5 in, 1 out]
      n101 = Index Array(array=w259, index=0 ("索引")) -> (element=w256:sgl)
      n102 = Subtract(x=sgl 360.0, y=w242) -> (x-y=w243:sgl)
      n103 = Less?(x=w256, y=w242) -> (x < y?=w255:bool)
      n104 = Greater?(x=w256, y=w243) -> (0:w254:bool)
      n105 = Or(x=w255, y=w254) -> (x .or. y?=w253:bool)
      n106 = case shown="真" w253 {
        tunnel: w236 -> [_ w479]
        tunnel: w235 -> [_ w478]
        tunnel: w234 -> [_ w477]
        tunnel: w233 -> [_ w476]
        tunnel: w249 -> [w266 w471]
        tunnel: [w266 w269] -> w260
        tunnel: w252 -> [w265 w472]
        tunnel: [w265 w381] -> w251
        tunnel: w250 -> [_ w464]
        tunnel: [FALSE w352] -> w241
        tunnel: w240 -> [_ w301]
        tunnel: [dbl[] [] ("Particle Measurements (Pixels) (Particle Analysis 1)") w348] -> w239
        tunnel: w238 -> [_ w304]
        tunnel: w237 -> [_ w312]
        tunnel: [FALSE w271] -> w232
        frame False {
        }
        frame True {
          w324 = cluster{"X":sgl, "Y":sgl} {"X"=-0.5, "Y"=-0.5}  # 第二点向胶木方向延伸比例
          w298 = "HXQGWDJ_ROIs" ("字符串")
          w369 = "HXQGWDJ_MASK" ("字符串")
          w413 = 0.18  # 扩展的槽区矩形半宽比例
          w414 = 0.1  # 槽区矩形半长比例
          w423 = sgl -0.3 ("X")
          w425 = sgl 0.5 ("X")
          w430 = 0.05  # 槽区矩形半宽比例
          w429 = 0.15  # 槽区矩形半长比例
          w407 = T26 {"Left"=0, "Top"=0, "Right"=0, "Bottom"=0, "Rotation"=0.0} ("Rectangle")
          w437 = cluster{"X":sgl, "Y":sgl} {"X"=1.0, "Y"=0.0}  # 构造X轴向
          w326 = cluster{"X":sgl, "Y":sgl} {"X"=0.0, "Y"=0.0}  # 第一点向铜底方向延伸比例
          w450 = T27 2 items=["弧度输入，弧度输出", "弧度输入，角度输出", "角度输入，角度输出", "角度输入，弧度输出"] ("angle units")
          w463 = 5.0 ("y")
          # "采用槽中线位于铜胶分界上的点作为基准，投影到原有半径上，重新计算偏移量"
          # "中心向底部方向适当偏移"
          # "这么繁琐的计算过程的原因是避免像素坐标的取整误差\n这个误差此处可能引入较大偏差"
          # "也可以通过测算，选择距离底部中点较近的点作为角度测量第三点"
          # "中分线端点远近次序不定，此处判断是否需要调序"
          n107 = Bundle("Point1 (Pixels)"=w479, "Point2 (Pixels)"=w478) -> (w475:T28)  [unwired: 1 in]
          n108 = Bundle("Point1 (Pixels)"=w477, "Point2 (Pixels)"=w476) -> (w474:T28)  [unwired: 1 in]
          n109 = call "IMAQ Bisecting Line"("error in (no error)"=w472, "Line 2"=w474, "Line 1"=w475) -> ("error out"=w400:errorcluster, "Bisecting Line"=w473:T29)  [unwired: 7 in]
          n110 = Random Number (0-1)() -> (number: 0 to 1=w399:dbl)
          n111 = Unbundle(w473) -> ("Point 1"=w457:cluster{"X":sgl, "Y":sgl}, "Point 2"=w456:cluster{"X":sgl, "Y":sgl})
          n112 = disable-structure shown="禁用" {
            disable-tunnel: w471 -> [w569 w576 w577]
            disable-tunnel: w457 -> [w565 w574 _]
            disable-tunnel: w456 -> [w564 w573 _]
            disable-tunnel: [w563 w575 w577] -> w331
            frame Disabled {
              n113 = Build Array(w565) -> (w570:cluster{"X":sgl, "Y":sgl}[])
              n114 = call "Overlay Feature Points.vi"("Color"=u32 6618880, "Feature Points"=w570, "Image"=w569) -> ("Image Out"=w567:T8)  [unwired: 7 in, 1 out]
              n115 = Build Array(w564) -> (w566:cluster{"X":sgl, "Y":sgl}[])
              n116 = call "Overlay Feature Points.vi"("Color"=u32 16750634, "Feature Points"=w566, "Image"=w567) -> ("Image Out"=w563:T8)  [unwired: 7 in, 1 out]
            }
            frame Disabled {
              n117 = call "IMAQ Overlay Line"("Color"=u32 9567230, "End Point"=w573, "Start Point"=w574, "Image"=w576) -> ("Image Out"=w575:T8)  [unwired: 6 in, 1 out]
            }
            frame Enabled {
            }
          }
          n118 = Multiply(x=w399, y=100000000.0) -> (x*y=w397:dbl)
          n119 = To Unsigned Long Integer(number=w397) -> (unsigned 32bit integer=w390:u32)
          n120 = Add(x=w457, y=cluster{"X":sgl, "Y":sgl} {"X"=1.0, "Y"=0.0}) -> (x+y=w468:cluster{"X":sgl, "Y":sgl})
          n121 = Increment(x=w390) -> (x+1=w384:u32)
          n122 = Build Array(w468, w456) -> (w467:cluster{"X":sgl, "Y":sgl}[])
          n123 = Number To Hexadecimal String(2:w390) -> (0:w396:string)  [unwired: 1 in]
          n124 = Increment(x=w384) -> (x+1=w370:u32)
          n125 = call "IMAQ Get Angles"("Vertex"=w457, "Points"=w467, "Use Vertex (No)"=TRUE) -> ("Angles (deg)"=w466:sgl[])  [unwired: 2 in, 2 out]
          n126 = Number To Hexadecimal String(2:w384) -> (0:w391:string)  [unwired: 1 in]
          n127 = Increment(x=w370) -> (x+1=w371:u32)
          n128 = Increment(x=w370) -> (x+1=w332:u32)
          n129 = Number To Hexadecimal String(2:w370) -> (0:w386:string)  [unwired: 1 in]
          n130 = Index Array(array=w466, index=0 ("索引")) -> (element=w459:sgl)
          n131 = Add(x=w464, y=w463) -> (x+y=w461:dbl)
          n132 = Increment(x=w332) -> (x+1=w297:u32)
          n133 = Number To Hexadecimal String(2:w371) -> (0:w372:string)  [unwired: 1 in]
          n134 = Subtract(x=w464, y=w463) -> (x-y=w462:dbl)
          n135 = Number To Hexadecimal String(2:w332) -> (0:w374:string)  [unwired: 1 in]
          n136 = Subtract(x=360.0, y=w459) -> (x-y=w458:dbl)
          n137 = Increment(x=w297) -> (x+1=w296:u32)
          n138 = Number To Hexadecimal String(2:w297) -> (0:w334:string)  [unwired: 1 in]
          n139 = call-poly <vilib>:"Check for Included Angle.vi"("angle units"=w450, "end angle"=w461, "start angle"=w462, "angle in"=w458) -> ("in range?"=w455:bool)  [unwired: 5 in, 2 out]
          "所得中线的端点属于正序" <- w455
          n140 = Concatenate Strings(w369, w396) -> (w395:string)
          n141 = Concatenate Strings(w369, w391) -> (w392:string)
          n142 = Concatenate Strings(w369, w386) -> (w385:string)
          n143 = Concatenate Strings(w369, w372) -> (w373:string)
          n144 = Unbundle(w457) -> ("X"=w454:sgl, "Y"=w453:sgl)
          n145 = Unbundle(w456) -> ("X"=w452:sgl, "Y"=w451:sgl)
          n146 = Number To Hexadecimal String(2:w296) -> (0:w299:string)  [unwired: 1 in]
          n147 = case shown="真" w455 {
            tunnel: w454 -> [w581 w585]
            tunnel: [w579 w585] -> w449
            tunnel: [w578 w584] -> w448
            tunnel: w453 -> [w580 w584]
            tunnel: [w581 w583] -> w447
            tunnel: w452 -> [w579 w583]
            tunnel: [w580 w582] -> w446
            tunnel: w451 -> [w578 w582]
            frame False {
            }
            frame True {
            }
          }
          n148 = call "IMAQ Create"("Image Name"=w395) -> ("New Image"=w359:T8)  [unwired: 4 in, 1 out]
          n149 = call "IMAQ Create"("Image Name"=w392) -> ("New Image"=w361:T8)  [unwired: 4 in, 1 out]
          n150 = call "IMAQ Create"("Image Name"=w385) -> ("New Image"=w382:T8)  [unwired: 4 in, 1 out]
          n151 = call "IMAQ Create"("Image Name"=w373) -> ("New Image"=w362:T8)  [unwired: 4 in, 1 out]
          n152 = Bundle "计算偏移"("X"=w423, "X"=w423) -> (w422:cluster{"X":sgl, "X":sgl})  [unwired: 1 in]
          n153 = Bundle("X"=w449, "Y"=w448) -> (w428:cluster{"X":sgl, "Y":sgl})  [unwired: 1 in]
          n154 = Bundle("X"=w447, "Y"=w446) -> (w318:cluster{"X":sgl, "Y":sgl})  [unwired: 1 in]
          n155 = Concatenate Strings(w298, w374) -> (w375:string)
          n156 = Concatenate Strings(w298, w334) -> (w333:string)
          n157 = Concatenate Strings(w298, w299) -> (w300:string)
          n158 = Add(x=w437, y=w428) -> (x+y=w438:cluster{"X":sgl, "Y":sgl})
          n159 = call "IMAQ Create"("Image Name"=w375) -> ("New Image"=w358:T8)  [unwired: 4 in, 1 out]
          n160 = call "IMAQ Create"("Image Name"=w333) -> ("New Image"=w321:T8)  [unwired: 4 in, 1 out]
          n161 = call "IMAQ Create"("Image Name"=w300) -> ("New Image"=w293:T8)  [unwired: 4 in, 1 out]
          n162 = Subtract(x=w428, y=w318) -> (x-y=w325:cluster{"X":sgl, "Y":sgl})
          n163 = Bundle "计算中点"("X"=w425, "X"=w425) -> (w424:cluster{"X":sgl, "X":sgl})  [unwired: 1 in]
          n164 = Add(x=w428, y=w318) -> (x+y=w427:cluster{"X":sgl, "Y":sgl})
          n165 = property on="边沿检测LineProfile原始" class="WFChart (严格)"("History Data"=dbl[] [] ("历史数据")) -> (error out=w329:errorcluster)  [unwired: 2 in, 1 out]
          n166 = Multiply(x=w325, y=w326) -> (x*y=w445:cluster{"X":sgl, "Y":sgl})
          n167 = Multiply(x=w325, y=w324) -> (x*y=w319:cluster{"X":sgl, "Y":sgl})
          n168 = Multiply ("x")(x=w325, y=w422) -> (x*y=w421:cluster{"X":sgl, sgl})
          n169 = Multiply "取中点"(x=w427, y=w424) -> (x*y=w426:cluster{"X":sgl, sgl})
          n170 = Add(x=w428, y=w445) -> (x+y=w444:cluster{"X":sgl, "Y":sgl})
          n171 = Build Array(w438, w318) -> (w439:cluster{"X":sgl, "Y":sgl}[])
          n172 = Add(x=w318, y=w319) -> (x+y=w317:cluster{"X":sgl, "Y":sgl})
          n173 = disable-structure shown="禁用" {
            disable-tunnel: w444 -> [w541 _]
            disable-tunnel: w318 -> [w540 _]
            disable-tunnel: w331 -> [w538 w542]
            disable-tunnel: [w537 w542] -> w314
            frame Disabled {
              n174 = call "IMAQ Overlay Line"("Color"=u32 9567230, "End Point"=w541, "Start Point"=w540, "Image"=w538) -> ("Image Out"=w537:T8)  [unwired: 6 in, 1 out]
            }
            frame Enabled {
            }
          }
          n175 = Add(x=w426, y=w421) -> (x+y=w420:cluster{"X":sgl, sgl})
          n176 = call "IMAQ Get Angles"("Vertex"=w428, "Points"=w439, "Use Vertex (No)"=TRUE) -> ("Angles (deg)"=w440:sgl[])  [unwired: 2 in, 2 out]
          n177 = Unbundle(w317) -> ("X"=w316:sgl, "Y"=w315:sgl)
          n178 = call "IMAQ GetImageSize"("Image"=w331) -> ("X Resolution"=w406:i32)  [unwired: 3 in, 2 out]
          n179 = Multiply(x=w406, y=w414) -> (x*y=w412:dbl)
          n180 = Multiply(x=w406, y=w413) -> (x*y=w416:dbl)
          n181 = Multiply(x=w406, y=w429) -> (x*y=w431:dbl)
          n182 = Multiply(x=w406, y=w430) -> (x*y=w417:dbl)
          n183 = Unbundle(w420) -> ("X"=w405:sgl, w404:sgl)
          n184 = Unbundle(w444) -> ("X"=w337:sgl, "Y"=w336:sgl)
          n185 = call "胶木二值图"("Image In"=w331, "Image Dst"=w321, "error in"=w329) -> ("Image Out"=w330:T8, "error out"=w328:errorcluster)  [unwired: 23 in]
          n186 = Index Array(array=w440, index=0 ("索引")) -> (element=w443:sgl)
          n187 = Add(x=w405, y=w412) -> (x+y=w410:dbl)
          n188 = Add(x=w405, y=w431) -> (x+y=w433:dbl)
          n189 = Subtract(x=w405, y=w412) -> (x-y=w408:dbl)
          n190 = Subtract(x=w405, y=w431) -> (x-y=w435:dbl)
          n191 = Bundle(cluster=T21 {"Start X"=0, "Start Y"=0, "End X"=0, "End Y"=0} ("Line"), "Start X"=w337, "Start Y"=w336, "End X"=w316, "End Y"=w315) -> (w346:T21)
          n192 = Subtract(x=360.0, y=w443) -> (x-y=w289:dbl)
          n193 = call "IMAQ Convert Line to ROI"("Line"=w346) -> ("ROI Descriptor"=w320:T14)  [unwired: 8 in, 1 out]
          n194 = Subtract(x=w404, y=w416) -> (x-y=w409:dbl)
          n195 = Add(x=w404, y=w416) -> (x+y=w411:dbl)
          n196 = Subtract(x=w404, y=w417) -> (x-y=w434:dbl)
          n197 = Add(x=w404, y=w417) -> (x+y=w432:dbl)
          n198 = call "IMAQ Edge Tool 3"("Image"=w330, "Edge Options"="溢槽槽向边沿检测", "Optimized Mode"=FALSE, "ROI Descriptor"=w320, "Process"=T13."Get First Edge", "error in (no error)"=w328) -> ("Image (duplicate)"=w308:T8, "Edge Information"=w340:T16[], "Gradient Values"=→"边沿检测LineProfile原始":dbl[])  [unwired: 5 in, 2 out]
          n199 = Bundle By Name "制作搜边选框"(cluster=w407, "Left"=w435, "Top"=w434, "Right"=w433, "Bottom"=w432, "Rotation"=w289) -> (w419:T26)
          n200 = Bundle By Name "制作搜边选框"(cluster=w407, "Left"=w408, "Top"=w409, "Right"=w410, "Bottom"=w411, "Rotation"=w289) -> (w415:T26)
          n201 = Index Array(array=w340, index=0 ("索引")) -> (element=w338:T16)
          n202 = call "IMAQ Convert Rectangle to ROI (Polygon)"("Rectangle"=w419) -> ("ROI Descriptor"=w393:T14)  [unwired: 7 in, 2 out]
          n203 = Unbundle By Name(w338) -> ("Location (Pixel)"=w310:cluster{"X":sgl, "Y":sgl})  [unwired: 1 out]
          n204 = call "IMAQ Convert Rectangle to ROI (Polygon)"("Rectangle"=w415) -> ("ROI Descriptor"=w389:T14)  [unwired: 7 in, 2 out]
          n205 = call "IMAQ Overlay ROI"("Colors (Green)"=u32[] [3381759], "ROI Descriptor"=w320, "Image"=w314) -> ("Image Out"=w323:T8)  [unwired: 7 in, 1 out]
          n206 = Bundle(w304, w312) -> (w311:cluster{cluster{dbl, dbl}, cluster{sgl, sgl}})  [unwired: 1 in]
          n207 = call "IMAQ Perpendicular Line"("Point"=w310, "Line"=w311) -> ("Perpendicular Line"=w309:T29)  [unwired: 7 in, 2 out]
          n208 = Unbundle By Name(w309) -> ("Point 2"=w305:cluster{"X":sgl, "Y":sgl})
          n209 = Build Array(w305) -> (w344:cluster{"X":sgl, "Y":sgl}[])
          n210 = Build Array(w304, w305) -> (w306:cluster{"X":dbl, "Y":dbl}[])
          n211 = call "Overlay Feature Points.vi"("Color"=u32 16776770, "Feature Points"=w344, "Image"=w323) -> ("Image Out"=w313:T8)  [unwired: 7 in, 1 out]
          n212 = call "IMAQ Point Distances"("Points"=w306) -> ("Distances"=w307:sgl[])  [unwired: 4 in, 1 out]
          n213 = Index Array(array=w307) -> (element=w303:sgl)  [unwired: 1 in]
          n214 = call "IMAQ Overlay ROI"("Colors (Green)"=u32[] [16738816], "error in (no error)"=w400, "ROI Descriptor"=w393, "Image"=w313) -> ("error out"=w401:errorcluster, "Image Out"=w402:T8)  [unwired: 6 in]
          n215 = Select(t=w301, s=FALSE, f=w303) -> (s? t:f=w291:sgl)
          n216 = call "IMAQ Overlay ROI"("Colors (Green)"=u32[] [14429696], "error in (no error)"=w401, "ROI Descriptor"=w389, "Image"=w402) -> ("error out"=w394:errorcluster, "Image Out"=w270:T8)  [unwired: 6 in]
          n217 = Subtract ("扣除截取半径与实际半径的差异")(x="偏移_顶洞_向上部修正量", y=w291) -> (x-y=w290:dbl)
          n218 = Subtract ("扣除截取半径与实际半径的差异")(x="偏移_钩端_向上部修正量", y=w291) -> (x-y=w351:dbl)
          n219 = call "tt-构建扇形ROI-A型式.vi"("R_ROI小圆半径"="R_顶洞检测小圆半径", "开启调试显示"=TRUE, "钩端向上部偏移量"=w290, "镜像产品角度"=w289, "扇形半张角"="ROI_顶洞检测扇形半张角", "ImageSrc"=w270) -> ("anROI"=w268:T14, "输出RECT"=w272:T22, "ImgOut"=→"ImgOut":T8)  [unwired: 2 in, 1 out]
          n220 = call "阈值处理"("Image In"=w270, "Image Dst"=w358) -> ("Image Out"=w357:T8)  [unwired: 24 in, 1 out]
          n221 = call "tt-构建扇形ROI-A型式.vi"("开启调试显示"=TRUE, "钩端向上部偏移量"=w351, "镜像产品角度"=w289, "ImageSrc"=w270) -> ("anROI"=w368:T14)  [unwired: 4 in, 3 out]
          n222 = call "顶洞二值图"("Image In"=w270, "Image Dst"=w293) -> ("Image Out"=w286:T8, "error out"=w285:errorcluster)  [unwired: 24 in]
          n223 = call "IMAQ ROIToMask 2"("Background Value (0)"=255, "Image Model"=w357, "error in (no error)"=w394, "Filling Value (255)"=0, "ROI Descriptor"=w393, "Image"=w359) -> ("error out"=w377:errorcluster, "Image Out"=w378:T8)  [unwired: 3 in, 1 out]
          n224 = call "IMAQ ROIToMask 2"("Image Model"=w357, "error in (no error)"=w377, "ROI Descriptor"=w389, "Image"=w361) -> ("error out"=w383:errorcluster, "Image Out"=w379:T8)  [unwired: 5 in, 1 out]
          n225 = call "IMAQ Multiply"("Image Src A"=w286, "Constant"=200.0, "error in (no error)"=w285) -> ("Image Dst Out"=w283:T8, "error out"=w282:errorcluster)  [unwired: 4 in]
          n226 = call "IMAQ Mask"("error in (no error)"=w383, "Image Dst"=w382, "Image Mask"=w378, "Image Src"=w379) -> ("error out"=w366:errorcluster, "Image Dst Out"=w376:T8)  [unwired: 1 in]
          n227 = call "IMAQ Find Circular Edge 3"("Circle Fit Options"="顶洞_Circle Fit Options", "Options"="顶洞_Options", "error in (no error)"=w282, "ROI Descriptor"=w268, "Image"=w283) -> ("error out"=w273:errorcluster, "Fitted Circle"=w277:T5, "Image Out"=w276:T8, "Circle Found"=w278:bool)  [unwired: 2 in, 1 out]
          "Fitted Circle" <- w277
          n228 = call "IMAQ ROIToMask 2"("Image Model"=w357, "error in (no error)"=w366, "ROI Descriptor"=w368, "Image"=w362) -> ("error out"=w365:errorcluster, "Image Out"=w364:T8)  [unwired: 5 in, 1 out]
          n229 = case shown="真" w278 {
            tunnel: w277 -> [_ w489]
            tunnel: w276 -> [_ w486]
            tunnel: w273 -> [w480 w485]
            tunnel: w272 -> [_ w490]
            tunnel: [FALSE w491] -> w271
            tunnel: w270 -> [w481 w488]
            tunnel: [w481 w487] -> w269
            tunnel: w268 -> [_ w484]
            tunnel: [w480 w483] -> w267
            frame False {
            }
            frame True {
              n230 = Unbundle By Name(w489) -> ("Radius (Pixels)"=w494:dbl)
              "顶洞圆半径" <- w494
              n231 = disable-structure shown="禁用" {
                disable-tunnel: w490 -> [w518 _]
                disable-tunnel: w489 -> [w517 _]
                disable-tunnel: w488 -> [w514 w536]
                disable-tunnel: [w513 w536] -> w487
                disable-tunnel: w486 -> [w502 _]
                disable-tunnel: w485 -> [w501 w535]
                disable-tunnel: w484 -> [w498 _]
                disable-tunnel: [w495 w535] -> w483
                frame Disabled {
                  w524 = 10.0 ("y")
                  n232 = Unbundle By Name(w517) -> ("Center (Pixels).X"=w519:sgl, "Center (Pixels).Y"=w520:sgl, "Radius (Pixels)"=w523:dbl)
                  n233 = Unbundle By Name(w518) -> ("Start Angle"=w515:dbl, "End Angle"=w516:dbl)
                  n234 = Subtract(x=w523, y=w524) -> (x-y=w522:dbl)
                  n235 = Add(x=w523, y=w524) -> (x+y=w521:dbl)
                  n236 = Bundle By Name(cluster=T22 {"Center X"=0, "Center Y"=0, "Inner Radius"=0, "Outer Radius"=0, "Start Angle"=0.0, "End Angle"=0.0} ("输出簇"), "Center X"=w519, "Center Y"=w520, "Start Angle"=w515, "End Angle"=w516, "Inner Radius"=w522, "Outer Radius"=w521) -> (w525:T22)
                  n237 = call "IMAQ Convert Annulus to ROI"("Annulus"=w525) -> ()  [unwired: 8 in, 2 out]
                  n238 = disable-structure shown="禁用" {
                    disable-tunnel: w502 -> [w532 w534]
                    disable-tunnel: w501 -> [w531 w533]
                    disable-tunnel: [w530 w534] -> w500
                    disable-tunnel: [w529 w533] -> w499
                    disable-tunnel: w498 -> [w527 _]
                    frame Disabled {
                      n239 = call "IMAQ Overlay ROI"("Colors (Green)"=u32[] [16730130], "error in (no error)"=w531, "ROI Descriptor"=w527, "Image"=w532) -> ("error out"=w529:errorcluster, "Image Out"=w530:T8)  [unwired: 6 in]
                    }
                    frame Enabled {
                    }
                  }
                  n240 = call "IMAQ Extract Contour"("Source Image"=w500, "Curve Extraction"="Curve Extraction Settings", "ROI Descriptor"=w498, "Search Direction"=T25."Annulus Outer To Inner", "error in (no error)"=w499, "Contour Selection"=T24."Maximum Length", "Curve Connection"=T23[] [{"Match Constraints"=0, "Min"=0.0, "Max"=25.0}, {"Match Constraints"=1, "Min"=0.0, "Max"=180.0}, {"Match Constraints"=2, "Min"=0.0, "Max"=25.0}, {"Match Constraints"=3, "Min"=0.0, "Max"=180.0}]) -> ("Source Image Out"=w511:T8, "error out"=w509:errorcluster)  [unwired: 1 in, 6 out]
                  n241 = call "IMAQ Compute Curvature"("error in (no error)"=w509, "Kernel Width"="Kernel Width", "Contour Image"=w511) -> ("error out"=w496:errorcluster, "Curvature Profile (pixel)"=→"Curvature Profile":dbl[], "Contour Image Out (dup)"=w497:T8)  [unwired: 6 out]
                  n242 = disable-structure shown="禁用" {
                    disable-tunnel: w497 -> [w526 _]
                    frame Disabled {
                      n243 = call "Vision Assistant3"("Image In"=w526) -> ()  [unwired: 25 in, 2 out]
                    }
                    frame Enabled {
                    }
                  }
                  n244 = call "IMAQ Overlay Contour"("error in (no error)"=w496, "Contour Points Settings"="Contour Points Settings", "Contour Image"=w497, "Image"=w514) -> ("error out"=w495:errorcluster, "Image Out"=w513:T8)  [unwired: 2 in, 4 out]
                }
                frame Enabled {
                }
              }
              n245 = In Range and Coerce(upper limit="顶洞圆半径上限", x=w494, lower limit="顶洞圆半径下限") -> (In Range?=w491:bool)  [unwired: 1 out]
              "顶洞圆半径正常" <- w491
            }
          }
          n246 = call "IMAQ Mask"("error in (no error)"=w365, "Image Dst"=w359, "Image Mask"=w376, "Image Src"=w357) -> ("error out"=w360:errorcluster, "Image Dst Out"=w367:T8)  [unwired: 1 in]
          n247 = call "IMAQ Mask"("error in (no error)"=w360, "Image Mask"=w364, "Image Src"=w367) -> ("error out"=w354:errorcluster, "Image Dst Out"=w356:T8)  [unwired: 2 in]
          n248 = call "分析颗粒"("Image In"=w356, "error in"=w354) -> ("Image Out"=w355:T8, "Number of Particles (Particle Analysis 1)"=w353:i32, "Particle Measurements (Pixels) (Particle Analysis 1)"=w349:dbl[][], "error out"=w274:errorcluster)  [unwired: 22 in]
          n249 = Equal To 0?(x=w353) -> (x = 0?=w352:bool)
          n250 = Empty Array?(array=w349) -> (empty?=w350:bool)
          n251 = case shown="假" w350 {
            tunnel: w349 -> [w545 _]
            tunnel: [w543 dbl[] [] ("Particle Measurements (Pixels) (Particle Analysis 1)")] -> w348
            frame False {
              n252 = Index Array(array=w545, index (row)=0 ("索引 (行)")) -> (element=w543:dbl[])  [unwired: 1 in]
            }
            frame True {
            }
          }
          n253 = Merge Errors(w267, w274) -> (w275:errorcluster)
          n254 = flat-sequence {
            tunnel: w275 -> [w547]
            tunnel: [w547] -> w380
            tunnel: w355 -> [_]
            tunnel: w359 -> [w562]
            tunnel: w361 -> [w561]
            tunnel: w382 -> [w560]
            tunnel: [w549] -> w381
            tunnel: w380 -> [w551]
            tunnel: w362 -> [w555]
            tunnel: w358 -> [w554]
            tunnel: w308 -> [w552]
            tunnel: w293 -> [w548]
            frame #0 {
            }
            frame #1 {
              n255 = call "IMAQ Dispose"("Image"=w562, "error in (no error)"=w551) -> ("error out"=w559:errorcluster)  [unwired: 4 in]
              n256 = call "IMAQ Dispose"("Image"=w561, "error in (no error)"=w559) -> ("error out"=w558:errorcluster)  [unwired: 4 in]
              n257 = call "IMAQ Dispose"("Image"=w560, "error in (no error)"=w558) -> ("error out"=w556:errorcluster)  [unwired: 4 in]
              n258 = call "IMAQ Dispose"("Image"=w555, "error in (no error)"=w556) -> ("error out"=w557:errorcluster)  [unwired: 4 in]
              n259 = call "IMAQ Dispose"("Image"=w554, "error in (no error)"=w557) -> ("error out"=w553:errorcluster)  [unwired: 4 in]
              n260 = call "IMAQ Dispose"("Image"=w552, "error in (no error)"=w553) -> ("error out"=w550:errorcluster)  [unwired: 4 in]
              n261 = call "IMAQ Dispose"("Image"=w548, "error in (no error)"=w550) -> ("error out"=w549:errorcluster)  [unwired: 4 in]
            }
          }
        }
      }
    }
    frame True {
    }
  }
  "ImageOUT" <- w164
  "error out" <- w165
  "钩外多胶正常" <- w90
  n262 = disable-structure shown="禁用" {
    frame Disabled {
    }
    frame Enabled {
    }
  }
  n263 = disable-structure shown="禁用" {
    disable-tunnel: _ -> [w609 _]
    disable-tunnel: [w608 _] -> _
    disable-tunnel: _ -> [w604 _]
    disable-tunnel: _ -> [w596 _]
    disable-tunnel: _ -> [w594 _]
    frame Disabled {
      w598 = 5.0 ("y")
      w612 = u16 0 items=["Outside To Inside", "Inside To Outside"] ("Scan Direction")
      n264 = Unbundle By Name(w609) -> ("Center (Pixels).X"=w606, "Center (Pixels).Y"=w605, "Radius (Pixels)"=w599)
      n265 = Unbundle By Name(w604) -> ("Start Angle"=w603, "End Angle"=w602)
      n266 = Subtract(x=w599, y=w598) -> (x-y=w600:dbl)
      n267 = Add(x=w599, y=w598) -> (x+y=w601:dbl)
      n268 = Bundle By Name(cluster=T22 {"Center X"=0, "Center Y"=0, "Inner Radius"=0, "Outer Radius"=0, "Start Angle"=0.0, "End Angle"=0.0} ("Annulus 2"), "Center X"=w606, "Center Y"=w605, "Start Angle"=w603, "End Angle"=w602, "Inner Radius"=w600, "Outer Radius"=w601) -> (w597:T22)
      n269 = call "IMAQ Convert Annulus to ROI"("Annulus"=w597) -> ("ROI Descriptor"=w593:T14)  [unwired: 8 in, 1 out]
      n270 = call "IMAQ Overlay ROI"("Colors (Green)"=u32[] [10813184], "error in (no error)"=w596, "ROI Descriptor"=w593, "Image"=w594) -> ("error out"=w595:errorcluster, "Image Out"=w591:T8)  [unwired: 6 in]
      n271 = call "IMAQ Spoke 4"("Image"=w591, "Edge Options"="顶洞_RakeEdge Options 2", "ROI Descriptor"=w593, "Scan Direction"=w612, "error in (no error)"=w595, "Process"=T13."Get First Edge") -> ("error out"=w608:errorcluster)  [unwired: 6 in, 3 out]
    }
    frame Enabled {
    }
  }
  n272 = disable-structure shown="禁用" {
    frame Disabled {
      n273 = call "Vision Assistant2"() -> ()  [unwired: 26 in, 2 out]
    }
    frame Enabled {
    }
  }
  n274 = disable-structure shown="禁用" {
    disable-tunnel: _ -> [w623 _]
    disable-tunnel: _ -> [w622 _]
    disable-tunnel: _ -> [w621 _]
    disable-tunnel: _ -> [w620 _]
    disable-tunnel: _ -> [w614 _]
    disable-tunnel: [w613 _] -> _
    frame Disabled {
      w615 = u32 16738816 ("Text Color (black)")
      n275 = call "IMAQ Overlay Text"("Text Color (black)"=w615, "String"="1", "Origin"=w623, "Image"=w614) -> ("Image Out"=w626:T8)  [unwired: 6 in, 1 out]
      n276 = call "IMAQ Overlay Text"("Text Color (black)"=w615, "String"="2", "Origin"=w622, "Image"=w626) -> ("Image Out"=w625:T8)  [unwired: 6 in, 1 out]
      n277 = call "IMAQ Overlay Text"("Text Color (black)"=w615, "String"="3", "Origin"=w621, "Image"=w625) -> ("Image Out"=w624:T8)  [unwired: 6 in, 1 out]
      n278 = call "IMAQ Overlay Text"("Text Color (black)"=w615, "String"="4", "Origin"=w620, "Image"=w624) -> ("Image Out"=w613:T8)  [unwired: 6 in, 1 out]
    }
    frame Enabled {
    }
  }
  n279 = Index Array(array="Global Rectangle", index #1=0 ("索引"), index #2=1 ("索引")) -> (element #1=w99:i32, element #2=w98:i32)
  n280 = Bundle(w99, w98, w99, w98) -> (w93:cluster{i32, i32, i32, i32})  [unwired: 1 in]
  n281 = case shown="假" w1 {
    selector: w1 -> [w627 w628]
    tunnel: [w627 w628] -> _
    frame False {
    }
    frame True {
    }
  }
  n282 = Index Array(array=w97, index #1=0 ("索引"), index #2=1 ("索引"), index #3=2 ("索引"), index #4=3 ("索引")) -> (element #1=w107:dbl, element #2=w106:dbl, element #3=w105:dbl, element #4=w104:dbl)
  n283 = Bundle("Numeric"=w107, "Numeric"=w106, "Numeric"=w105, "Numeric"=w104) -> (w92:T9)  [unwired: 1 in]
  "多胶异常RECT本地" <- w92
  n284 = case shown="假" w90 {
    selector: w90 -> [w629 w630]
    tunnel: [w629 w630] -> _
    frame False {
    }
    frame True {
    }
  }
  n285 = Add(x=w92, y=w93) -> (x+y=→"多胶异常RECT":cluster{dbl, dbl, dbl, dbl})
  n286 = disable-structure shown="禁用" {
    disable-tunnel: _ -> [w631 _]
    frame Disabled {
      n287 = call "Vision Assistant"("Image In"=w631) -> ()  [unwired: 25 in, 2 out]
    }
    frame Enabled {
    }
  }
  "顶洞缺胶状态正常" <- w1
